vi "Update Fan.vi"(8 "error in (no error)":errorcluster, 9 "Fan B":cluster{"State":bool, "Fault":bool}, 10 "Fan A":cluster{"State":bool, "Fault":bool}, 11 "Cooler UI in":refnum<class "Cooler UI with Events.lvclass">=refnum) -> (0 "error out":errorcluster, 3 "Cooler UI out":refnum<class "Cooler UI with Events.lvclass">)   [LabVIEW 2012, in "Cooler UI.lvlib" / "Cooler UI with Events.lvclass"]
uses:
  Cooler UI with Events.lvclass
  Cooler UI with Events.lvclass/Cooler UI with Events.ctl
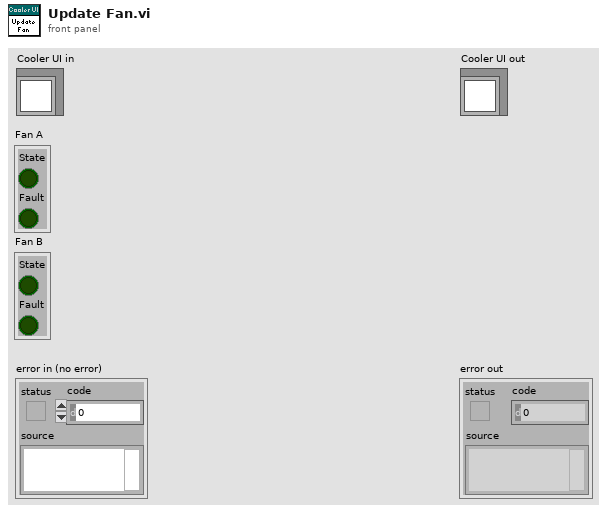
[diagram p1: front panel]
types:
  T1 = cluster{"Fan A":cluster{"State":bool, "Fault":bool}, "Fan B":cluster{"State":bool, "Fault":bool}}
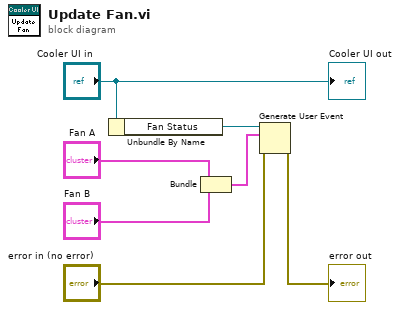
[diagram p0: block diagram]
diagram:
  n1 = Unbundle By Name("Cooler UI in") -> ("Fan Status"=w7:refnum<user-event>)
  n2 = Bundle("Fan A"="Fan A", "Fan B"="Fan B") -> (w4:T1)  [unwired: 1 in]
  n3 = Generate User Event(user event=w7, event data cluster=w4, error in="error in (no error)") -> (error out=→"error out":errorcluster)  [unwired: 1 out]
  "Cooler UI out" <- "Cooler UI in"
